vi "getCategoriesLikeName.vi"(8 "error in (no error)":errorcluster, 10 "Name filter":string, 11 "Database in":refnum<class "Account History.lvclass">) -> (0 "error out":errorcluster, 2 "CategoryList out":refnum<class "CategoryList.lvclass">, 3 "Database out":refnum<class "Account History.lvclass">)   [LabVIEW 2018, in "Account History.lvclass"]
uses:
  Account History.lvclass
  CategoryList/CategoryList.lvclass
  Category/Category.lvclass
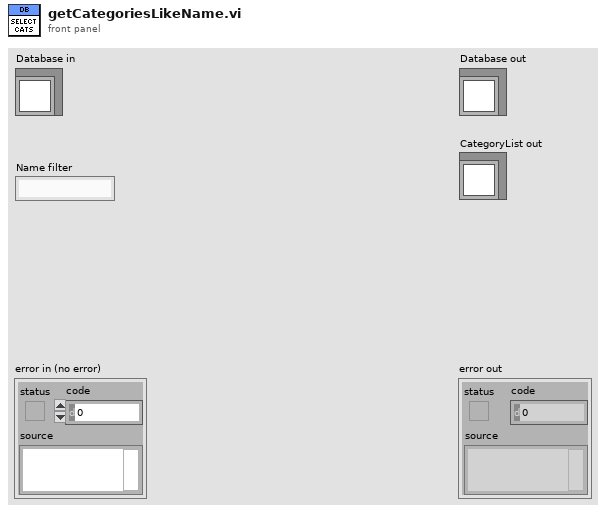
[diagram p1: front panel]
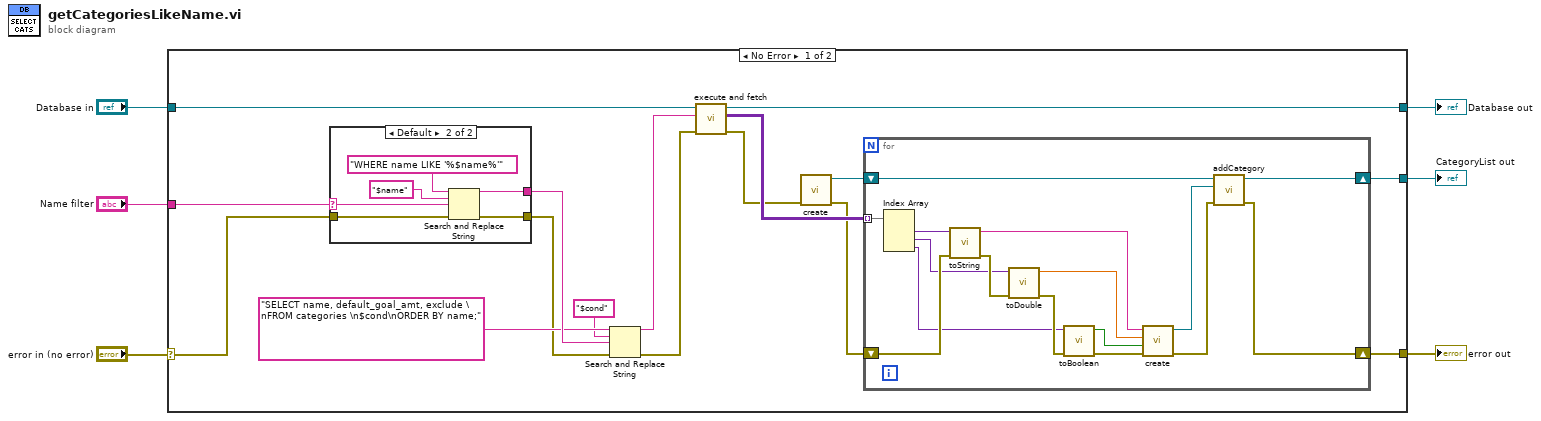
[diagram p0: block diagram]
diagram:
  n1 = case shown="No Error" "error in (no error)" {
    selector: "error in (no error)" -> [w12 w46]
    tunnel: [w16 w47] -> w6
    tunnel: "Database in" -> [w15 w47]
    tunnel: [w14 w46] -> w4
    tunnel: "Name filter" -> [w13 _]
    tunnel: [w7 _] -> w1
    frame No Error {
      n2 = case shown="Default" w13 {
        selector: w13 -> [_ w29]
        tunnel: [_ w26] -> w20
        tunnel: w12 -> [w23 w25]
        tunnel: [w23 w24] -> w11
        frame "" {
        }
        frame Default {
          n3 = Search and Replace String(input string="WHERE name LIKE '%$name%'", search string="$name", replace string=w29, error in=w25) -> (result string=w26:string, error out=w24:errorcluster)  [unwired: 4 in, 2 out]
        }
      }
      n4 = Search and Replace String(input string="SELECT name, default_goal_amt, exclude \nFROM categories \n$cond\nORDER BY name;", search string="$cond", replace string=w20, error in=w11) -> (result string=w17:string, error out=w21:errorcluster)  [unwired: 4 in, 2 out]
      n5 = call "execute and fetch.vi"("error in (no error)"=w21, "SQL query"=w17, "Database in"=w15) -> ("error out"=w9:errorcluster, "recordset data"=w22:variant[][], "Database out"=w16:refnum<class "Account History.lvclass">)  [unwired: 5 in, 1 out]
      n6 = call "create.vi"("error in (no error)"=w9) -> ("error out"=w8:errorcluster, "CategoryList out"=w10:refnum<class "CategoryList.lvclass">)  [unwired: 9 in]
      n7 = for {
        tunnel: w22 -> [w45] mode=indexing
        shift-right: [w39] -> w14
        shift-left: w8 -> [w38]
        shift-right: [w42] -> w7
        shift-left: w10 -> [w43]
        n8 = Index Array(array=w45) -> (element #1=w37:variant, element #2=w36:variant, element #3=w32:variant)  [unwired: 3 in]
        n9 = call "toString.vi"("error in (no error)"=w38, "Variant"=w37) -> ("error out"=w44:errorcluster, "String"=w35:string)  [unwired: 8 in]
        n10 = call "toDouble.vi"("error in (no error)"=w44, "Value"=w36) -> ("error out"=w33:errorcluster, "type"=w34:dbl)  [unwired: 8 in]
        n11 = call "toBoolean.vi"("error in (no error)"=w33, "Variant"=w32) -> ("error out"=w31:errorcluster, "Boolean"=w30:bool)  [unwired: 8 in]
        n12 = call "create.vi"("error in (no error)"=w31, "Exclude"=w30, "Default Goal Amount"=w34, "Name"=w35) -> ("error out"=w40:errorcluster, "Category out"=w41:refnum<class "Category.lvclass">)  [unwired: 6 in]
        n13 = call "addCategory.vi"("error in (no error)"=w40, "Category.lvclass"=w41, "CategoryList in"=w43) -> ("error out"=w39:errorcluster, "CategoryList out"=w42:refnum<class "CategoryList.lvclass">)  [unwired: 7 in]
      }
    }
    frame Error {
    }
  }
  "error out" <- w4
  "Database out" <- w6
  "CategoryList out" <- w1
